vi "IMU_Read_SENSOR.vi"(7 "Sensors Present":u16[](array[numeric]), 8 "error in (no error)":errorcluster caption="Fehler (Eingang, kein Fehler)", 10 "VISA resource name IN":refnum<visa-resource-name>, 11 "MultiWii Data Cluster 2":refnum<vi>) -> (0 "error out":errorcluster caption="Fehler (Ausgang)", 2 "VISA resource name OUT":refnum<visa-resource-name>)   [LabVIEW 2017]
uses:
  IMU_Data_Cluster.ctl
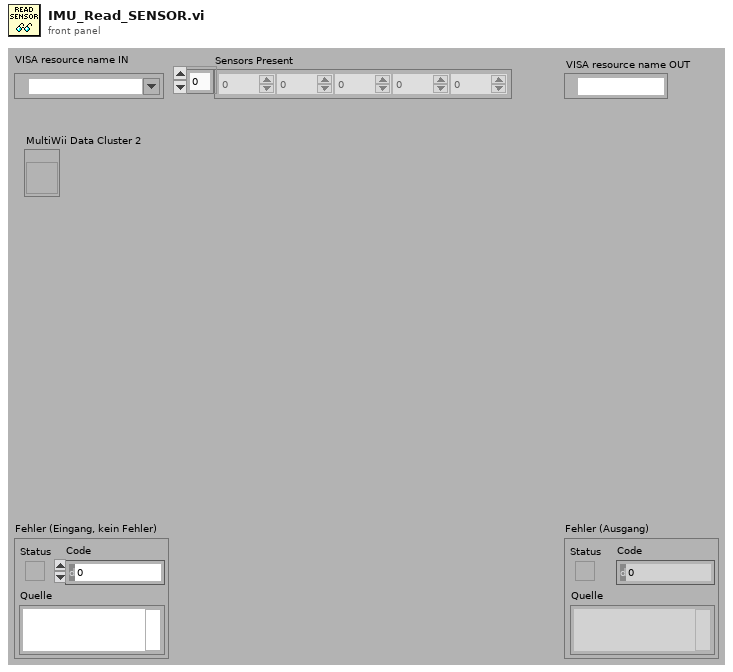
[diagram p1: front panel]
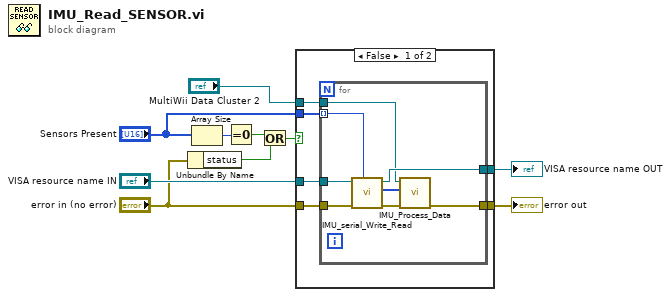
[diagram p0: block diagram]
diagram:
  n1 = Unbundle By Name("error in (no error)") -> ("status"=w5:bool)
  n2 = Array Size(array="Sensors Present") -> (size(s)=w4:i32)
  n3 = Equal To 0?(x=w4) -> (x = 0?=w3:bool)
  n4 = Or(x=w3, y=w5) -> (x .or. y?=w6:bool)
  n5 = case shown="False" w6 {
    tunnel: "error in (no error)" -> [w15 w25]
    tunnel: "VISA resource name IN" -> [w16 w26]
    tunnel: [w14 w26] -> w9
    tunnel: [w13 w25] -> w8
    tunnel: "Sensors Present" -> [w12 _]
    tunnel: "MultiWii Data Cluster 2" -> [w11 _]
    frame False {
      n6 = for {
        tunnel: w12 -> [w22] mode=indexing
        tunnel: w16 -> [w21]
        tunnel: w15 -> [w20]
        tunnel: [w19] -> w14
        tunnel: [w18] -> w13
        tunnel: w11 -> [w17]
        n7 = call "IMU_serial_Write_Read.vi"("Command Selection"=w22, "error in (no error)"=w20, "VISA resource name IN"=w21) -> ("error IO"=w24:errorcluster, "Received Raw Data Byte-Array U8"=w23:u8[], "VISA resource name OUT"=w19:refnum<visa-resource-name>)  [unwired: 6 in]
        n8 = call "IMU_Process_Data.vi"("error in (no error)"=w24, "Received Raw Data Byte-Array U8"=w23, "MultiWii Data Cluster 2"=w17) -> ("error out"=w18:errorcluster)  [unwired: 8 in]
      }
    }
    frame True {
    }
  }
  "VISA resource name OUT" <- w9
  "error out" <- w8
